vi "Demo.vi"() -> ()   [LabVIEW 2022 SP3, in "Core.lvlib"]
uses:
  Core.lvlib
panel:
  out "ID out":i32
  out "Parent ID":i32
  out "Name":string
  in  "Toggle Tool Bar":bool
  in  "Toggle Menu Bar":bool
  in  "Show Diagram":bool
  out "Time":timestamp format="%<%H:%M:%S%3u>T"
  in  "UI Exit":bool
  out "Config Section":string
  out "Config Path":path
  in  "ID":i32
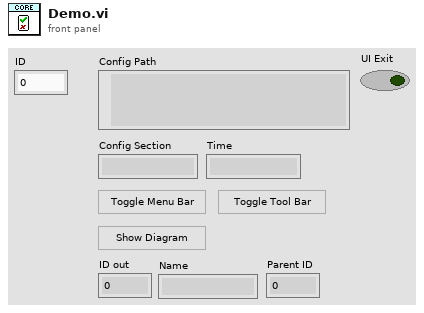
[diagram p1: front panel]
types:
  T1 = typedef "Core.lvlib/Module.ctl" = cluster{"ID":i32, "Name":string, "Parent ID":i32, "Instance":refnum<data-value>, "Self":T2}
  T2 = typedef "Core.lvlib/Module Instance.ctl" = cluster{"Queue":refnum<queue>, "Config Path":path, "Config Section":string}
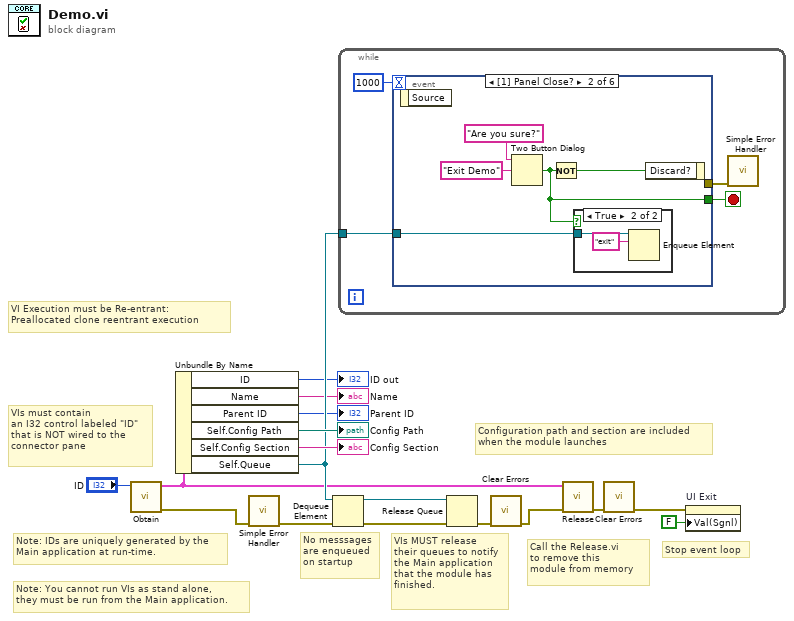
[diagram p0: block diagram]
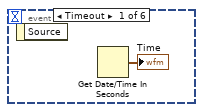
[diagram p2: hidden frame]
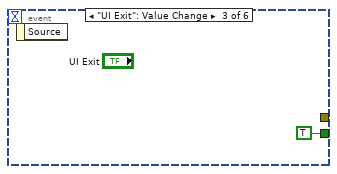
[diagram p4: hidden frame]
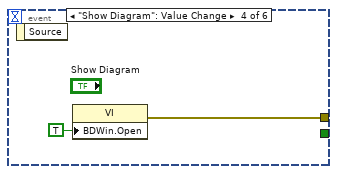
[diagram p5: hidden frame]
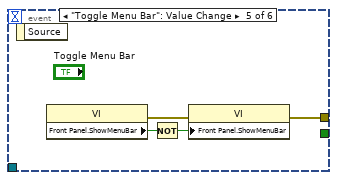
[diagram p6: hidden frame]
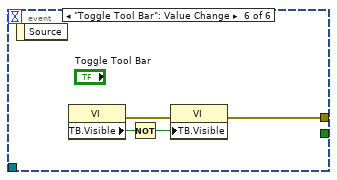
[diagram p7: hidden frame]
diagram:
  # "Note: IDs are uniquely generated by the\nMain application at run-time."
  # "Note: You cannot run VIs as stand alone,\nthey must be run from the Main application."
  # "Configuration path and section are included\nwhen the module launches"
  # "Call the Release.vi\nto remove this\nmodule from memory"
  # "Stop event loop"
  # "VIs MUST release\ntheir queues to notify\nthe Main application\nthat the module has\nfinished."
  # "No messsages\nare enqueued\non startup"
  # "VI Execution must be Re-entrant:\nPreallocated clone reentrant execution"
  # "VIs must contain\nan I32 control labeled \"ID\"\nthat is NOT wired to the\nconnector pane"
  n1 = call "Obtain.vi"("ID"="ID") -> ("error out"=w2:errorcluster, "Module"=w6:T1)  [unwired: 9 in]
  n2 = Unbundle By Name(w6) -> ("ID"=→"ID out":i32, "Name"=→"Name":string, "Parent ID"=→"Parent ID":i32, "Self.Config Path"=→"Config Path":path, "Self.Config Section"=→"Config Section":string, "Self.Queue"=w13:refnum<queue>)
  n3 = call <vilib>:"Simple Error Handler.vi"("error in (no error)"=w2) -> ("error out"=w1:errorcluster)  [unwired: 4 in, 4 out]
  n4 = Dequeue Element(queue=w13, error in (no error)=w1) -> (queue out=w17:refnum<queue>, error out=w16:errorcluster)  [unwired: 1 in, 2 out]
  n5 = while {
    tunnel: w13 -> [w21]
    stop <- w20 stop-if-true
    n6 = event shown="[1] Panel Close?" {
      selector: _ -> [_ _ _ _ _ _]
      dyn-events: _ -> [_ _ _ _ _ _]
      timeout: 1000 -> [_ _ _ _ _ _]
      tunnel: w21 -> [_ w24 _ _ _ _]
      tunnel: [_ w23 TRUE ("T button?") _ _ _] -> w20
      tunnel: [_ _ _ w31 w33 w37] -> w18
      event Timeout {
        n7 = event-data() -> ()  [unwired: 1 in, 1 out]
        n8 = Get Date/Time In Seconds() -> (seconds since 1Jan1904=→"Time":timestamp)
      }
      event Panel Close? {
        n9 = event-data() -> ()  [unwired: 1 in, 1 out]
        n10 = Two Button Dialog(message="Are you sure?", 2:"Exit Demo" ("T button name (\"OK\")")) -> (T button?=w23:bool)  [unwired: 1 in]
        n11 = Not(x=w23) -> (.not. x?=w25:bool)
        n12 = case shown="True" w23 {
          tunnel: w24 -> [_ w29]
          frame False {
          }
          frame True {
            n13 = Enqueue Element(queue=w29, element="exit") -> ()  [unwired: 2 in, 3 out]
          }
        }
        n14 = event-data("Discard?"=w25) -> ()  [unwired: 1 in, 1 out]
      }
      event "UI Exit": Value Change {
        n15 = event-data() -> ()  [unwired: 1 in, 1 out]
      }
      event "Show Diagram": Value Change {
        n16 = event-data() -> ()  [unwired: 1 in, 1 out]
        n17 = property class="VI"("BDWin.Open"=TRUE ("Block Diagram Window:Open")) -> (error out=w31:errorcluster)  [unwired: 2 in, 1 out]
      }
      event "Toggle Menu Bar": Value Change {
        n18 = event-data() -> ()  [unwired: 1 in, 1 out]
        n19 = property class="VI"() -> (error out=w36:errorcluster, "Front Panel.ShowMenuBar"=w35:bool)  [unwired: 2 in, 1 out]
        n20 = Not(x=w35) -> (.not. x?=w34:bool)
        n21 = property class="VI"(error in=w36, "Front Panel.ShowMenuBar"=w34) -> (error out=w33:errorcluster)  [unwired: 1 in, 1 out]
      }
      event "Toggle Tool Bar": Value Change {
        n22 = event-data() -> ()  [unwired: 1 in, 1 out]
        n23 = property class="VI"() -> (error out=w40:errorcluster, "TB.Visible"=w39:bool)  [unwired: 2 in, 1 out]
        n24 = Not(x=w39) -> (.not. x?=w38:bool)
        n25 = property class="VI"(error in=w40, "TB.Visible"=w38) -> (error out=w37:errorcluster)  [unwired: 1 in, 1 out]
      }
    }
    n26 = call <vilib>:"Simple Error Handler.vi"("error in (no error)"=w18) -> ()  [unwired: 4 in, 5 out]
  }
  n27 = Release Queue(queue=w17, error in (no error)=w16) -> (error out=w12:errorcluster)  [unwired: 1 in, 2 out]
  n28 = call <vilib>:"Clear Errors.vi"("error in (no error)"=w12) -> ("error out"=w10:errorcluster)  [unwired: 5 in, 1 out]
  n29 = call "Release.vi"("error in (no error)"=w10, "Module"=w6) -> ("error out"=w8:errorcluster)  [unwired: 8 in, 1 out]
  n30 = call <vilib>:"Clear Errors.vi"("error in (no error)"=w8) -> ("error out"=w7:errorcluster)  [unwired: 5 in, 1 out]
  n31 = property on="UI Exit" class="Bool (strict)"(error in=w7, "Val(Sgnl)"=FALSE ("Value (Signaling)")) -> ()  [unwired: 1 in, 2 out]
